vi "Remove Line.vi"(8 "error in":errorcluster, 10 "Active Line Name":string, 11 "Objects":T1) -> (0 "error out":errorcluster)   [LabVIEW 2013, in "OPC UA editor node.lvclass"]
doc: "This VI will remove a line from the configuration and disconect any tag connected to the channels in the line"
uses:
  OPC UA editor node.lvclass
  <vilib>/NI/DCAF Table API/Table Manager/object ref.ctl
  <vilib>/NI/DCAF/Tag Editor Core/Configuration Editor/Classes/Engine Parent/Engine Parent Editor Node.lvclass
  <vilib>/NI/DCAF/Tag Editor Core/Configuration Editor/Classes/Module editor node/module editor node.lvclass
  module/configuration/OPC UA configuration.lvclass
  <vilib>/NI/Configuration Framework/serializable configuration/NISE_CEF_serializable configuration.lvclass/NISE_CEF_serializable configuration.ctl
  <vilib>/Utility/LVClass/Get LV Class Name.vi
  <vilib>/NI/Configuration Framework/error generator/NISE_error generator.vi
  <vilib>/NI/Configuration Framework/serializable configuration/NISE_CEF_serializable configuration.lvclass
  <vilib>/NI/DCAF Table API/Table Manager/Table Manager.lvclass
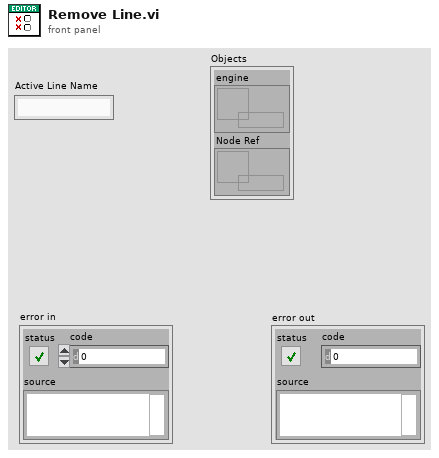
[diagram p1: front panel]
types:
  T1 = typedef "Table Manager.lvlib/Table Manager.lvclass/object ref.ctl" = cluster{"engine":refnum<data-value>, "Node Ref":refnum<data-value>}
  T2 = typedef "OPC UA configuration.lvclass/Line.ctl" = cluster{"channel":refnum<class "TBM channel.lvclass">, "Node Path":string, "OPC UA Data Type":enum16{"Bool", "SByte", "Byte", "Int16", "UInt16", "Int32", "UInt32", "Int64", "UInt64", "Float", "Double", "String", "DateTime", "ByteString", "Bool Array", "SByte Array", "Byte Array", "Int16 Array", "UInt16 Array", "Int32 Array", "UInt32 Array", "Int64 Array", "UInt64 Array", "Float Array", "Double Array", "String Array", "DateTime Array", "ByteString Array"}}
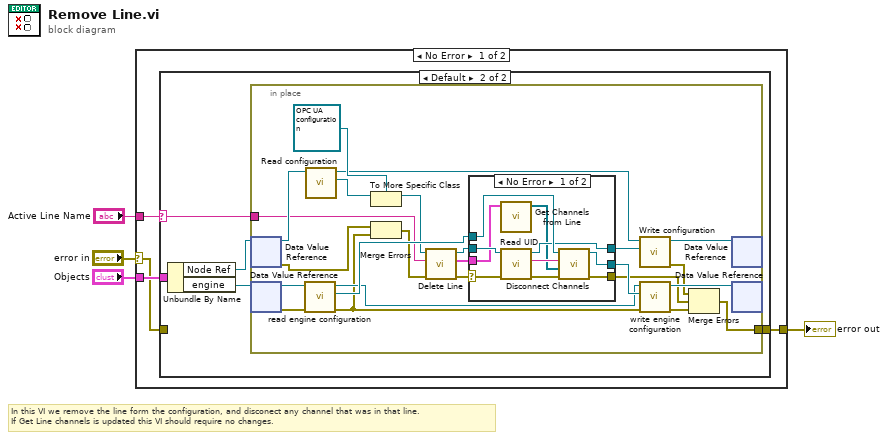
[diagram p0: block diagram]
diagram:
  # "In this VI we remove the line form the configuration, and disconect any channel that was in that line.\nIf Get Line channels is updated this VI should require no changes."
  n1 = case shown="No Error" "error in" {
    selector: "error in" -> [w5 w52]
    tunnel: "Objects" -> [w7 _]
    tunnel: [w8 w52] -> w3
    tunnel: "Active Line Name" -> [w6 _]
    frame No Error {
      n2 = case shown="Default" w6 {
        selector: w6 -> [_ w10]
        tunnel: [w9 w14] -> w8
        tunnel: w7 -> [_ w13]
        tunnel: w5 -> [w9 _]
        frame " " {
        }
        frame Default {
          n3 = Unbundle By Name(w13) -> ("Node Ref"=w11:refnum<data-value>, "engine"=w12:refnum<data-value>)
          n4 = in-place {
            in-place-border: [w17] -> w14
            in-place-border: w10 -> [w24]
            n5 = in-place-dvr #1(w11) -> (w30:refnum<class "module editor node.lvclass">, w31:errorcluster)
            n6 = in-place-dvr #2(w12) -> (w36:refnum<class "Engine Parent Editor Node.lvclass">, w35:errorcluster)
            n7 = call <vilib>:"read engine configuration.vi"("error in"=w35, "Engine Parent Editor Node in"=w36) -> ("error out"=w32:errorcluster, "engine configuration"=w34:refnum<class "engine configuration.lvclass">, "Engine Parent Editor Node out"=w33:refnum<class "Engine Parent Editor Node.lvclass">)  [unwired: 7 in]
            n8 = call-dynamic "Read configuration.vi"("NISE_CEF_serializable node in"=w30) -> ("configuration"=w28:refnum<class "NISE_CEF_serializable configuration.lvclass">, "NISE_CEF_serializable node out"=w26:refnum<class "module editor node.lvclass">)  [unwired: 8 in, 1 out]
            n9 = To More Specific Class(target class=refnum<class "OPC UA configuration.lvclass"> refnum ("tag bus configurable plugin module configuration out"), reference=w28) -> (specific class reference=w23:refnum<class "OPC UA configuration.lvclass">)  [unwired: 1 in, 1 out]
            n10 = Merge Errors(w31, w32) -> (w21:errorcluster)
            n11 = call "Delete Line.vi"("error in"=w21, "Active Line Name"=w24, "OPC UA configuration in"=w23) -> ("error out"=w20:errorcluster, "deleted line"=w15:T2, "OPC UA configuration out"=w22:refnum<class "OPC UA configuration.lvclass">)  [unwired: 6 in]
            n12 = case shown="No Error" w20 {
              selector: w20 -> [w42 w49]
              tunnel: w22 -> [w46 w50]
              tunnel: w34 -> [w48 w51]
              tunnel: [w47 w51] -> w37
              tunnel: [w43 w50] -> w25
              tunnel: [w41 w49] -> w16
              tunnel: w15 -> [w40 _]
              frame No Error {
                n13 = call "Get Channels from Line.vi"("Line"=w40) -> ("Array"=w39:refnum<class "TBM channel.lvclass">[])  [unwired: 10 in]
                n14 = call <vilib>:"Read UID.vi"("error in"=w42, "configuration in"=w46) -> ("error out"=w44:errorcluster, "instance id"=w45:string, "configuration out"=w43:refnum<class "OPC UA configuration.lvclass">)  [unwired: 7 in]
                n15 = call "Disconnect Channels.vi"("error in (no error)"=w44, "Deleted Channels"=w39, "instance id"=w45, "engine configuration in"=w48) -> ("error out"=w41:errorcluster, "engine configuration out"=w47:refnum<class "engine configuration.lvclass">)  [unwired: 6 in]
              }
              frame Error {
              }
            }
            n16 = call-dynamic "Write configuration.vi"("configuration"=w25, "NISE_CEF_serializable node in"=w26) -> ("error out"=w19:errorcluster, "NISE_CEF_serializable node out"=w27:refnum<class "module editor node.lvclass">)  [unwired: 8 in]
            n17 = call <vilib>:"write engine configuration.vi"("error in"=w32, "engine configuration"=w37, "Engine Parent Editor Node in"=w33) -> ("error out"=w18:errorcluster, "Engine Parent Editor Node out"=w38:refnum<class "Engine Parent Editor Node.lvclass">)  [unwired: 7 in]
            n18 = Merge Errors(w19, w16, w18) -> (w17:errorcluster)
            n19 = in-place-dvr #1(w27) -> ()  [unwired: 2 out]
            n20 = in-place-dvr #2(w38) -> ()  [unwired: 2 out]
          }
        }
      }
    }
    frame Error {
    }
  }
  "error out" <- w3
